vi "Write Header.vi"(8 "error in (no error)":errorcluster, 10 "operation (replace)":T1(ring)=enum."replace or create", 11 "Path":path) -> (0 "error out":errorcluster, 1 "IFD Offset Position":i64, 2 "Offset":i32=8, 3 "Byte Stream File out":refnum<file>, 4 "byte order (0:big-endian, network order)":T2(ring))   [LabVIEW 2020, in "LV Tiff.lvlib"]
uses:
  LV Tiff.lvlib
panel:
  out "Identifier":u16 format="%x"
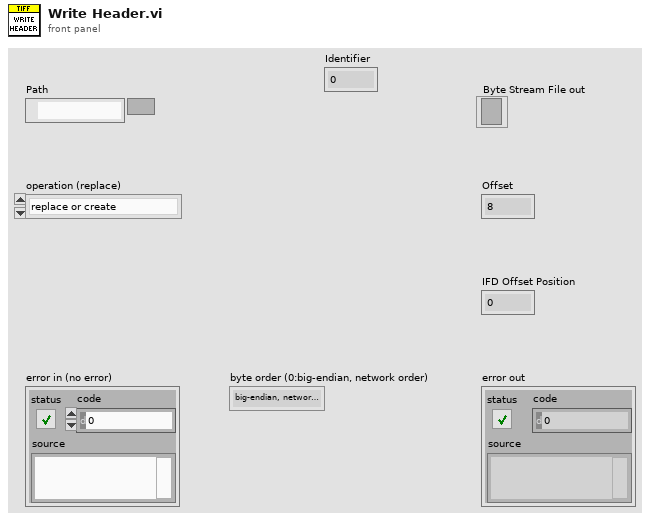
[diagram p1: front panel]
types:
  T1 = enum16{"open", "replace", "create", "open or create", "replace or create", "replace or create with confirmation"}
  T2 = enum16{"big-endian, network order", "native, host order", "little-endian"}
  T3 = cluster{"Identifier":u16, "Version":u16, "IFDOffset":u32}
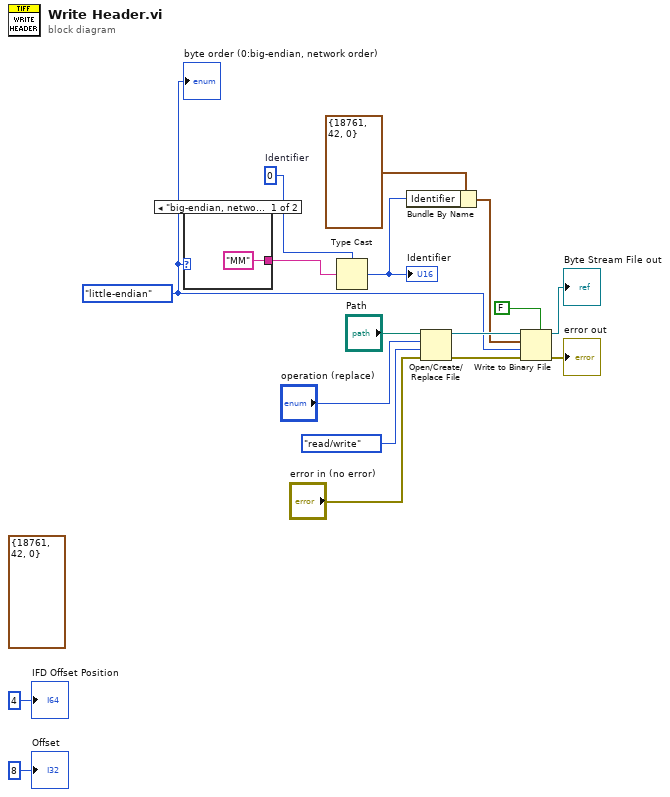
[diagram p0: block diagram]
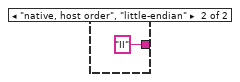
[diagram p2: hidden frame]
diagram:
  w1 = u16 0  # Identifier
  (unwired) T3 {"Identifier"=18761, "Version"=42, "IFDOffset"=0}
  w4 = T2."little-endian" ("byte order (0:big-endian, network order)")
  n1 = case shown="\"big-endian, network order\", Default" w4 {
    tunnel: ["MM" "II"] -> w3
    frame "big-endian, network order", Default {
    }
    frame "native, host order", "little-endian" {
    }
  }
  n2 = Type Cast(type=w1, x=w3) -> (*(type *) &x=w2:u16)
  "Identifier" <- w2
  n3 = Bundle By Name(cluster=T3 {"Identifier"=18761, "Version"=42, "IFDOffset"=0}, "Identifier"=w2) -> (w5:T3)
  n4 = Open/Create/Replace File(file path (use dialog)="Path", error in="error in (no error)", operation (0:open)="operation (replace)", access (0:read/write)=enum16{"read/write", "read-only", "write-only"}."read/write") -> (refnum out=w11:refnum<file>, error out=w10:errorcluster)  [unwired: 2 in, 1 out]
  n5 = Write to Binary File(file (use dialog)=w11, data=w5, error in=w10, 5:FALSE ("prepend array or string size? (T)"), 9:w4) -> (refnum out=→"Byte Stream File out":refnum<file>, error out=→"error out":errorcluster)  [unwired: 1 in, 1 out]
  "IFD Offset Position" <- i64 4 ("IFD Offset Position")
  "byte order (0:big-endian, network order)" <- w4
  "Offset" <- 8
